vi "Get Result.vi"   [LabVIEW 2014, in "Associated Power Technologies 8500 Series.lvlib"]
uses:
  <instrlib>/Associated Power Technologies 8500 Series/Associated Power Technologies 8500 Series.lvlib
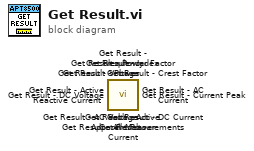
[diagram p0: block diagram]
diagram:
  n1 = call <instrlib>:"Get Result - Active Apparent Power.vi"() -> ()  [unwired: 13 in, 3 out]
  n2 = call <instrlib>:"Get Result - Crest Factor.vi"() -> ()  [unwired: 13 in, 3 out]
  n3 = call <instrlib>:"Get Result - Active Reactive Current.vi"() -> ()  [unwired: 13 in, 3 out]
  n4 = call <instrlib>:"Get Result - Current Peak.vi"() -> ()  [unwired: 13 in, 3 out]
  n5 = call <instrlib>:"Get Result - Power Factor.vi"() -> ()  [unwired: 13 in, 3 out]
  n6 = call <instrlib>:"Get Result - Power.vi"() -> ()  [unwired: 13 in, 3 out]
  n7 = call <instrlib>:"Get Result - DC Current.vi"() -> ()  [unwired: 13 in, 3 out]
  n8 = call <instrlib>:"Get Result - AC Current.vi"() -> ()  [unwired: 13 in, 3 out]
  n9 = call <instrlib>:"Get Result - Current.vi"() -> ()  [unwired: 13 in, 3 out]
  n10 = call <instrlib>:"Get Result - Frequency.vi"() -> ()  [unwired: 13 in, 3 out]
  n11 = call <instrlib>:"Get Result - DC Voltage.vi"() -> ()  [unwired: 13 in, 3 out]
  n12 = call <instrlib>:"Get Result - AC Voltage.vi"() -> ()  [unwired: 13 in, 3 out]
  n13 = call <instrlib>:"Get Result - Voltage.vi"() -> ()  [unwired: 13 in, 3 out]
  n14 = call <instrlib>:"Get Result - All Measurements.vi"() -> ()  [unwired: 13 in, 3 out]
  n15 = call <instrlib>:"Get Result - Index.vi"() -> ()  [unwired: 13 in, 3 out]
